vi "Add Frequency Measurement Channels.vi"(8 "error in (no error)":errorcluster, 9 "Frequency Measurement":T1[](array[typedef]) {"Edge" items=["Falling"=10171, "Rising"=10280]}, 11 "DAQ Ref":refnum<k24>) -> (0 "error out":errorcluster, 3 "DAQ Ref":refnum<k24>)   [LabVIEW 2019, in "Simple SysDef API.lvlib"]
uses:
  <userlib>/SimpleSysDef/Simple SysDef API.lvlib
  NationalInstruments.VeriStand.SystemDefinitionAPI
  <userlib>/SimpleSysDef/_SubVIs/Add Frequency Measurement Channels_Settings.ctl
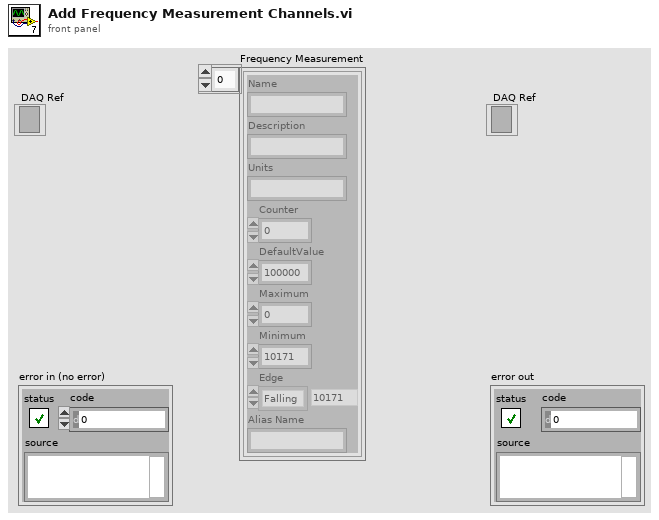
[diagram p1: front panel]
types:
  T1 = typedef "Simple SysDef API.lvlib/Add Frequency Measurement Channels_Settings.ctl" = cluster{"Name":string, "Description":string, "Units":string, "Counter":u32, "DefaultValue":dbl, "Maximum":dbl, "Minimum":dbl, "Edge":i32, "Alias Name":string}
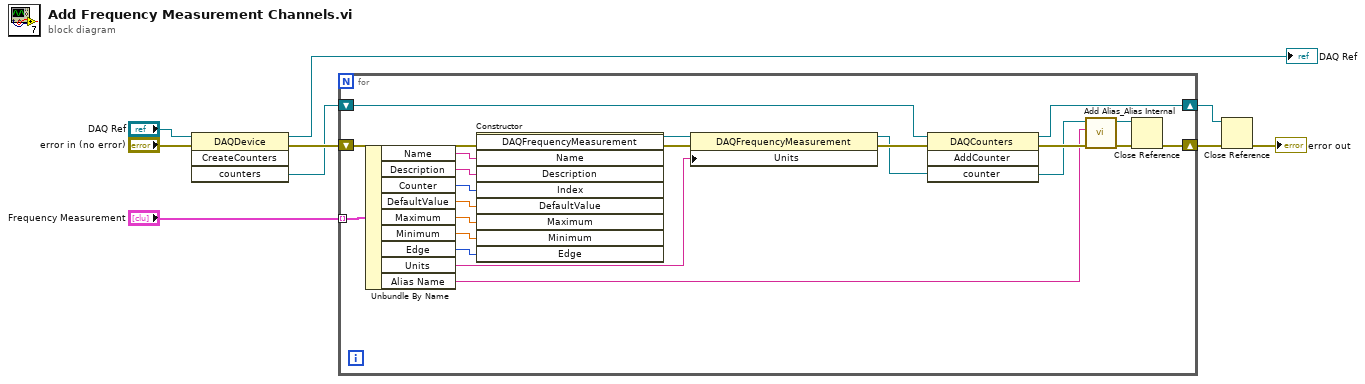
[diagram p0: block diagram]
diagram:
  n1 = invoke class="DAQDevice" method="CreateCounters"(reference="DAQ Ref", error in="error in (no error)") -> (reference out=→"DAQ Ref":refnum<k24>, error out=w4:errorcluster, "counters"=w3:refnum<k24>)  [unwired: 2 in, 1 out]
  n2 = for {
    shift-right: [w28] -> w6
    shift-left: w4 -> [w29]
    shift-right: [w27] -> w7
    shift-left: w3 -> [w30]
    tunnel: "Frequency Measurement" -> [w23] mode=indexing
    n3 = Unbundle By Name(w23) -> ("Name"=w22:string, "Description"=w21:string, "Counter"=w20:u32, "DefaultValue"=w19:dbl, "Maximum"=w18:dbl, "Minimum"=w17:dbl, "Edge"=w16:i32, "Units"=w15:string, "Alias Name"=w10:string)
    n4 = constructor class="DAQFrequencyMeasurement"(error in=w29, "Name"=w22, "Description"=w21, "Index"=w20, "DefaultValue"=w19, "Maximum"=w18, "Minimum"=w17, "Edge"=w16) -> (reference out=w26:refnum<k24>, error out=w25:errorcluster)  [unwired: 2 in, 8 out]
    n5 = property class="DAQFrequencyMeasurement"(reference=w26, error in=w25, "Units"=w15) -> (reference out=w12:refnum<k24>, error out=w24:errorcluster)
    n6 = invoke class="DAQCounters" method="AddCounter"(reference=w30, error in=w24, "counter"=w12) -> (reference out=w27:refnum<k24>, error out=w14:errorcluster)  [unwired: 1 in, 2 out]
    n7 = call <userlib>:"Add Alias_Alias Internal.vi"("error in (no error)"=w14, "Name"=w10, "Base Node"=w12) -> ("error out"=w13:errorcluster, "Base Node out"=w11:refnum<k24>)  [unwired: 7 in]
    n8 = Close Reference(reference=w11, error in (no error)=w13) -> (error out=w28:errorcluster)
  }
  n9 = Close Reference(reference=w7, error in (no error)=w6) -> (error out=→"error out":errorcluster)
